vi "to Time.vi"(8 "error in (no error)":errorcluster, 11 "time":T1) -> (0 "error out":errorcluster, 2 "time stamp":timestamp, 3 "time string":string)   [LabVIEW 2020]
uses:
  <vilib>/Utility/miscctls.llb/LVDateTimeRec.ctl
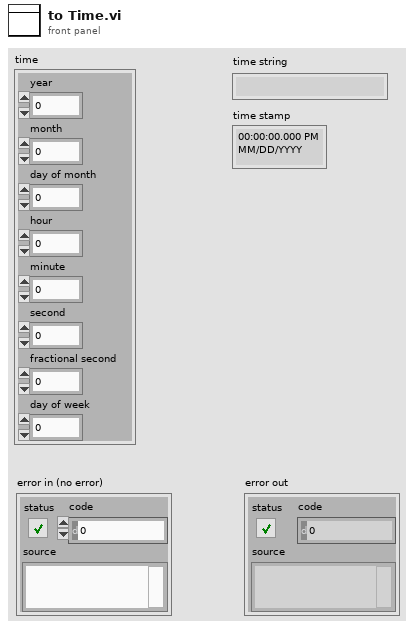
[diagram p1: front panel]
types:
  T1 = cluster{"year":u16, "month":u16, "day of month":u16, "hour":u16, "minute":u16, "second":u16, "fractional second":dbl, "day of week":u16}
  T2 = typedef "LVDateTimeRec.ctl" = cluster{"fractional second":dbl, "second":i32, "minute":i32, "hour":i32, "day of month":i32, "month":i32, "year":i32, "day of week":i32, "day of year":i32, "DST":i32}
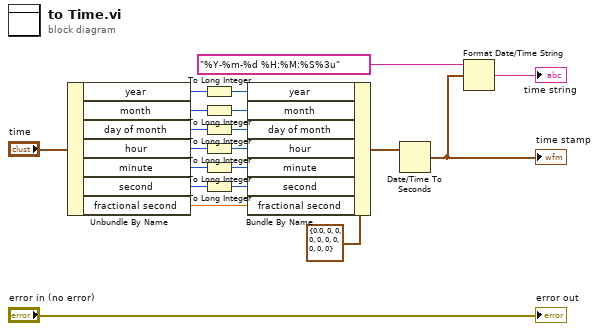
[diagram p0: block diagram]
diagram:
  n1 = Unbundle By Name("time") -> ("year"=w12:u16, "month"=w13:u16, "day of month"=w14:u16, "hour"=w15:u16, "minute"=w16:u16, "second"=w17:u16, "fractional second"=w18:dbl)
  n2 = To Long Integer(number=w12) -> (32bit integer=w6:i32)
  n3 = To Long Integer(number=w13) -> (32bit integer=w5:i32)
  n4 = To Long Integer(number=w14) -> (32bit integer=w4:i32)
  n5 = To Long Integer(number=w15) -> (32bit integer=w3:i32)
  n6 = To Long Integer(number=w16) -> (32bit integer=w2:i32)
  n7 = To Long Integer(number=w17) -> (32bit integer=w1:i32)
  n8 = Bundle By Name(cluster=T2 {"fractional second"=0.0, "second"=0, "minute"=0, "hour"=0, "day of month"=0, "month"=0, "year"=0, "day of week"=0, "day of year"=0, "DST"=0} ("date time rec"), "year"=w6, "month"=w5, "day of month"=w4, "hour"=w3, "minute"=w2, "second"=w1, "fractional second"=w18) -> (w11:T2)
  n9 = Date/Time To Seconds(2:w11) -> (0:w9:timestamp)  [unwired: 1 in]
  "time stamp" <- w9
  n10 = Format Date/Time String(time format string (%c)="%Y-%m-%d %H:%M:%S%3u" ("format string"), seconds (now)=w9) -> (date/time string=→"time string":string)  [unwired: 1 in]
  "error out" <- "error in (no error)"
